vi "sub_state-check_fgv.vi"(7 "cmd":enum16{"ini", "add", "use", "check"}(ring), 8 "error in":errorcluster) -> (0 "error out":errorcluster, 2 "element":string, 3 "data":bool)   [LabVIEW 2018]
panel:
  in  "item":string
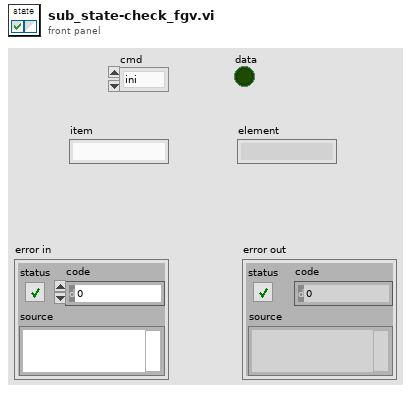
[diagram p1: front panel]
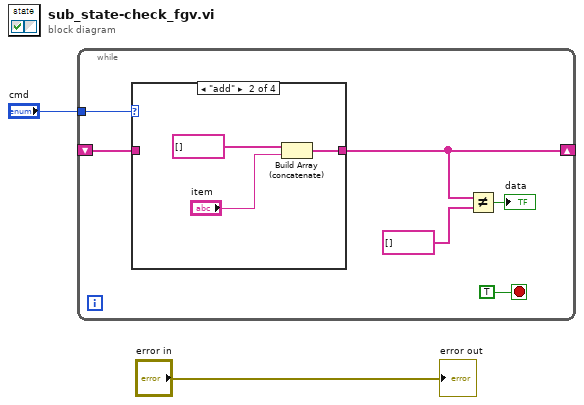
[diagram p0: block diagram]
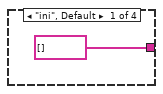
[diagram p2: hidden frame]
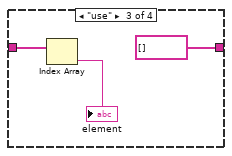
[diagram p3: hidden frame]
diagram:
  n1 = while {
    tunnel: "cmd" -> [w7]
    shift-right: [w5] -> _
    shift-left: _ -> [w6]
    stop <- TRUE stop-if-true
    n2 = case shown="\"add\"" w7 {
      tunnel: w6 -> [_ _ w15 w16]
      tunnel: [string[] [] w11 string[] [] w16] -> w5
      frame "ini", Default {
      }
      frame "add" {
        n3 = Build Array (concatenate)(string[] [], "item") -> (w11:string[])
      }
      frame "use" {
        n4 = Index Array(array=w15) -> (element=→"element":string)  [unwired: 1 in]
      }
      frame "check" {
      }
    }
    n5 = Not Equal?(x=w5, y=string[] []) -> (x != y?=→"data":bool)
  }
  "error out" <- "error in"
